vi "load_recipes.vi"(8 "error in (no error)":errorcluster, 11 "recipe":T2=enum."default") -> (0 "error out":errorcluster, 2 "transition []":string, 3 "recipe []":T1[](array[typedef]))   [LabVIEW 2015, in "example_02.lvlib"]
uses:
  example_02.lvlib
  _controls/recipes.ctl
  <userlib>/antonio-alexander/lv-recipe-machine/public/_controls/recipe_step.ctl
  _controls/steps_actions.ctl
  <userlib>/antonio-alexander/lv-recipe-machine/lv-recipe-machine.lvlib
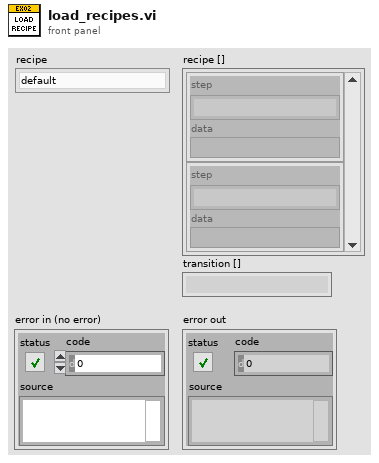
[diagram p1: front panel]
types:
  T1 = typedef "lv-recipe-machine.lvlib/recipe_step.ctl" = cluster{"step":string, "data":variant}
  T2 = typedef "example_02.lvlib/recipes.ctl" = enum16{"<recipes>", "default", "<null>"}
  T3 = typedef "example_02.lvlib/steps_actions.ctl" = enum16{"<steps_actions>", "auto_start", "auto_first_name", "auto_last_name", "auto_address", "auto_city", "auto_state", "auto_zip_code", "auto_submit", "auto_finish", "transition", "<null>"}
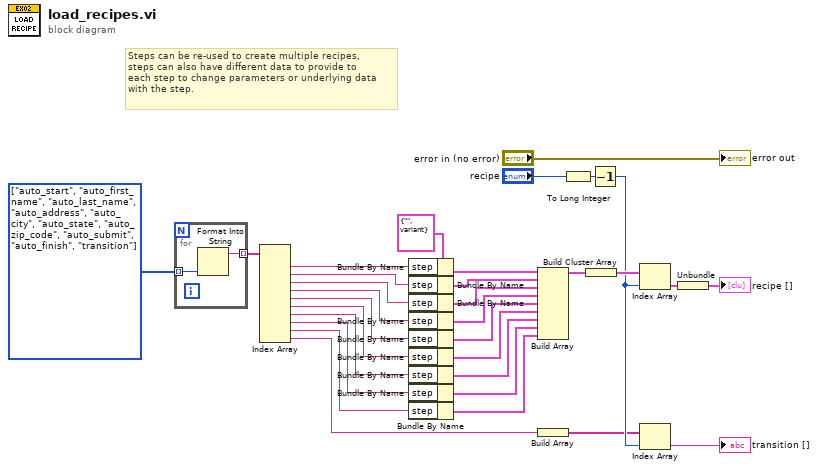
[diagram p0: block diagram]
diagram:
  w23 = T3[] [enum."auto_start", enum."auto_first_name", enum."auto_last_name", enum."auto_address", enum."auto_city", enum."auto_state", enum."auto_zip_code", enum."auto_submit", enum."auto_finish", enum."transition"] items=["<steps_actions>", "auto_start", "auto_first_name", "auto_last_name", "auto_address", "auto_city", "auto_state", "auto_zip_code", "auto_submit", "auto_finish", "transition", "<null>"]
  w3 = T1 {"step"="", "data"=variant} ("lv-recipe-machine.lvlib:recipe_step")
  # "Steps can be re-used to create multiple recipes,\nsteps can also have different data to provide to\neach step to change parameters or underlying data\nwith the step."
  n1 = for {
    tunnel: w23 -> [w34] mode=indexing
    tunnel: [w33] -> w22 mode=indexing
    n2 = Format Into String(w34) -> (resulting string=w33:string)  [unwired: 3 in, 1 out]
  }
  n3 = Index Array(array=w22) -> (element #1=w18:string, element #2=w17:string, element #3=w16:string, element #4=w14:string, element #5=w13:string, element #6=w12:string, element #7=w11:string, element #8=w5:string, element #9=w1:string, element #10=w4:string)  [unwired: 10 in]
  n4 = Bundle By Name(cluster=w3, "step"=w18) -> (w20:T1)
  n5 = Bundle By Name(cluster=w3, "step"=w17) -> (w19:T1)
  n6 = Bundle By Name(cluster=w3, "step"=w16) -> (w15:T1)
  n7 = Bundle By Name(cluster=w3, "step"=w14) -> (w10:T1)
  n8 = Bundle By Name(cluster=w3, "step"=w13) -> (w9:T1)
  n9 = Bundle By Name(cluster=w3, "step"=w12) -> (w8:T1)
  n10 = Bundle By Name(cluster=w3, "step"=w11) -> (w7:T1)
  n11 = Bundle By Name(cluster=w3, "step"=w5) -> (w6:T1)
  n12 = Bundle By Name(cluster=w3, "step"=w1) -> (w2:T1)
  n13 = Build Array(w20, w19, w15, w10, w9, w8, w7, w6, w2) -> (w24:T1[])
  n14 = Build Array(w4) -> (w21:string[])
  n15 = To Long Integer(number="recipe") -> (32bit integer=w29:i32)
  n16 = Build Cluster Array(w24) -> (w32:cluster{T1[]}[])
  n17 = Decrement(x=w29) -> (x-1=w26:i32)
  n18 = Index Array(array=w32, index=w26) -> (element=w28:cluster{T1[]})
  n19 = Index Array(array=w21, index=w26) -> (element=→"transition []":string)
  n20 = Unbundle(w28) -> (→"recipe []":T1[])
  "error out" <- "error in (no error)"
